vi "Save MATLAB File.vi"() -> ()   [LabVIEW 2020]
panel:
  in  "delimiter (Tab)":string
  out "spreadsheet string":string
  in  "base path":path
  in  "format string":string
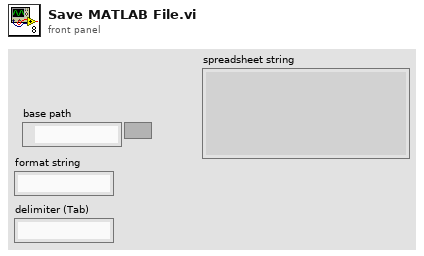
[diagram p1: front panel]
types:
  T1 = enum16{"open", "replace", "create", "open or create", "replace or create", "replace or create with confirmation"}
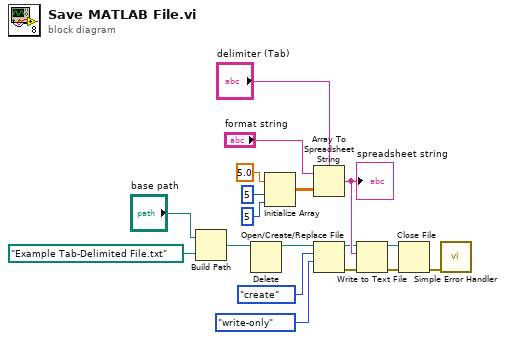
[diagram p0: block diagram]
diagram:
  n1 = Build Path(base path="base path", name or relative path=path "Example Tab-Delimited File.txt" ("default name")) -> (appended path=w8:path)
  n2 = Delete(path (use dialog)=w8) -> (deleted path=w6:path)  [unwired: 4 in, 2 out]
  n3 = Initialize Array(5.0 ("element"), 5 ("dimension size"), 5 ("dimension size")) -> (w13:dbl[][])
  n4 = Array To Spreadsheet String(delimiter (Tab)="delimiter (Tab)", array=w13, 3:"format string") -> (spreadsheet string=w12:string)
  "spreadsheet string" <- w12
  n5 = Open/Create/Replace File(file path (use dialog)=w6, operation (0:open)=T1."create", access (0:read/write)=enum16{"read/write", "read-only", "write-only"}."write-only") -> (refnum out=w5:refnum<file>, error out=w4:errorcluster)  [unwired: 1 in, 3 out]
  n6 = Write to Text File(file (use dialog)=w5, text=w12, error in=w4) -> (refnum out=w18:refnum<file>, error out=w17:errorcluster)  [unwired: 1 in, 1 out]
  n7 = Close File(refnum=w18, error in=w17) -> (error out=w3:errorcluster)  [unwired: 1 out]
  n8 = call <vilib>:"Simple Error Handler.vi"("error in (no error)"=w3) -> ()  [unwired: 1 in, 8 out]
